vi "Enqueue Message to Tx Command FIFO (Node).vi"(7 "Timeout":i32, 8 "error in":errorcluster, 9 "Input Valid":bool=TRUE, 10 "Command":T2, 11 "FIFOs: I/O Node":T1) -> (0 "error out":errorcluster, 1 "Success?":bool, 3 "FIFOs: I/O Node":T1)   [LabVIEW 2014, in "IO Node Logic Template_SPIBus1.lvlib"]
uses:
  IO Node Logic Template_SPIBus1.lvlib
  Controls/NodeResources FIFOs.ctl
  <vilib>/rvi/Emulation/niFpgaSctlEmulationGetInTimedLoop.vi
  <vilib>/rvi/DataTransferAndStorage/Container/Common/niFpgaContainerExecOnDevCompGetState.vi
  <vilib>/rvi/Emulation/niFpgaEmulationIsFPGAContextNoSignature.vi
  <vilib>/rvi/errors/niFpgaSetErrorForExecOnDevCompSimple.vi
  <vilib>/rvi/eio/common/nirviEmuReportErrorAndStop.vi
  <vilib>/rvi/DataTransferAndStorage/Container/Common/niFpgaContainerGetUniqueNameForEmu.vi
  <vilib>/rvi/FIFO/Fifo_Resource/nirvififoEmulationSetSize.vi
  <vilib>/rvi/FIFO/Fifo_Resource/nirviFifoEmulationQueueMgr.vi
  <instcachedir>/0/nirviFifoEmulationQueueMgr_E5CAEC123FF24DC58D834DCA3CDAA9B5.lvgen/nirviFifoEmulationQueueMgr_E5CAEC123FF24DC58D834DCA3CDAA9B5_001.vi
  <vilib>/rvi/FIFO/Fifo_Resource/nirvififoEmulationDetermineInputValidOut.vi
  <vilib>/rvi/FIFO/Fifo_Resource/nirvififoEmulationCreateLock.vi
  <vilib>/rvi/Emulation/niFpgaProcessEmulError.vi
  <vilib>/rvi/FIFO/Fifo_Resource/nirvififoEmulationObtainLock.vi
  <vilib>/rvi/FIFO/Fifo_Resource/nirvififoEmulationReleaseLock.vi
  <vilib>/rvi/occurrence/nirviWaitOnOccurrenceBase.vi
  <vilib>/rvi/errors/nirviReportUnexpectedCaseInternalError.vi
  <vilib>/rvi/errors/nirviReportUnexpectedCaseInternalError (U32).vi
  <vilib>/rvi/interface/RandomDataEmulation/niFpgaRandomDataHandleErrors.vi
  <vilib>/rvi/DataTransferAndStorage/Container/XNode/niFpgaContainer.xnode
  <vilib>/rvi/FIFO/Fifo_Resource/niFpgaFifoEmulationRefIn.vi
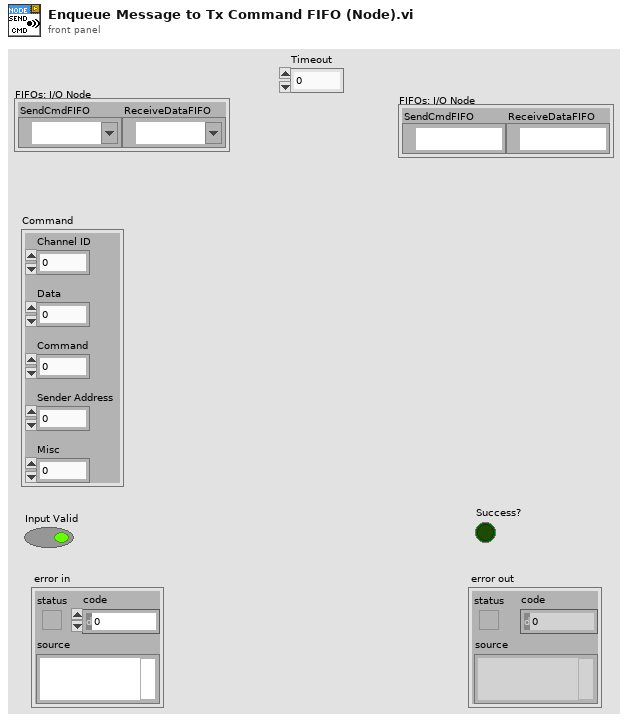
[diagram p1: front panel]
types:
  T1 = typedef "IO Node Logic Template_SPIBus1.lvlib/NodeResources FIFOs.ctl" = cluster{"SendCmdFIFO":refnum<k21>, "ReceiveDataFIFO":refnum<k21>}
  T2 = cluster{"Channel ID":u8, "Data":u64, "Command":u8, "Sender Address":u8, "Misc":u8}
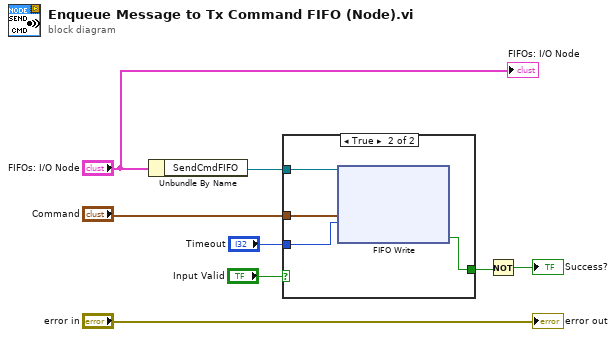
[diagram p0: block diagram]
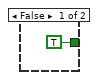
[diagram p2: hidden frame]
diagram:
  n1 = Unbundle By Name("FIFOs: I/O Node") -> ("SendCmdFIFO"=w4:refnum<k21>)
  n2 = case shown="True" "Input Valid" {
    tunnel: [TRUE ("Timed Out?") w13] -> w6
    tunnel: w4 -> [_ w12]
    tunnel: "Command" -> [_ w11]
    tunnel: "Timeout" -> [_ w10]
    frame False {
    }
    frame True {
      n3 = xnode "FIFO Write"("Element"=w11, "Timeout"=w10, "FIFO In"=w12) -> ("Timed Out?"=w13:bool)  [unwired: 1 out]
    }
  }
  n4 = Not(x=w6) -> (.not. x?=→"Success?":bool)
  "error out" <- "error in"
  "FIFOs: I/O Node" <- "FIFOs: I/O Node"
